vi "imageLocation.vi"(2 "extension":string="png", 3 "exposureTime":dbl, 4 "baseName":string="blah", 5 "basePath":path) -> (0 "imageLocation":path, 1 "imageLocationString":string)   [LabVIEW 2021]
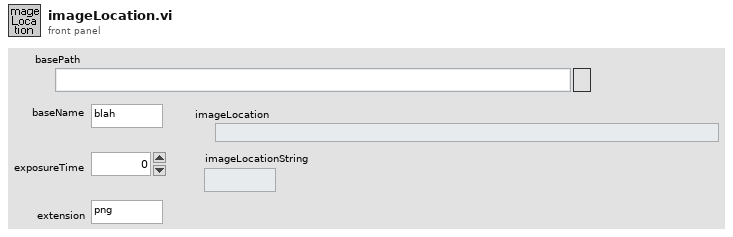
[diagram p1: front panel]
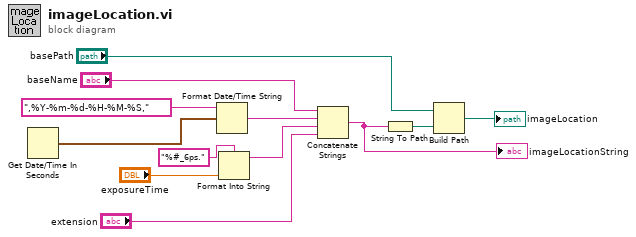
[diagram p0: block diagram]
diagram:
  n1 = Get Date/Time In Seconds() -> (seconds since 1Jan1904=w10:timestamp)
  n2 = Format Date/Time String(time format string (%c)=",%Y-%m-%d-%H-%M-%S,", seconds (now)=w10) -> (date/time string=w11:string)  [unwired: 1 in]
  n3 = Format Into String(format string="%#_6ps." ("initial string"), "exposureTime") -> (resulting string=w3:string)  [unwired: 2 in, 1 out]
  n4 = Concatenate Strings("baseName", w11, w3, "extension") -> (w5:string)
  "imageLocationString" <- w5
  n5 = String To Path(string=w5) -> (path=w7:path)
  n6 = Build Path(base path="basePath", name or relative path=w7) -> (appended path=→"imageLocation":path)
